vi "File Attachment Example.vi"() -> ()   [LabVIEW 2024]
uses:
  Sift API/Sift Client.lvclass
  Sift API/Types/Entity Type.ctl
  Sift Client.lvlib
panel:
  in  "Run Name":string
  out "Error":errorcluster
  in  "API Key":string
  in  "API URL":string
  # "Sift File Attachment Upload Example"
  # "Note: This example will not run as-is. \nOpen the VI to update the pathnames to valid files to run the example."
  # "Run this example to test uploading file attachments files to Sift."
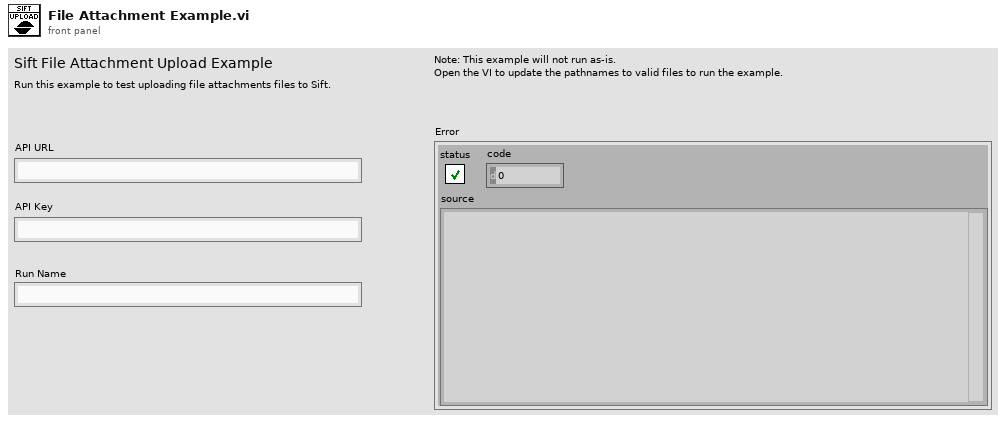
[diagram p1: front panel]
types:
  T1 = typedef "Sift Client.lvlib/Entity Type.ctl" = enum16{"runs", "annotations", "annotation_logs"}
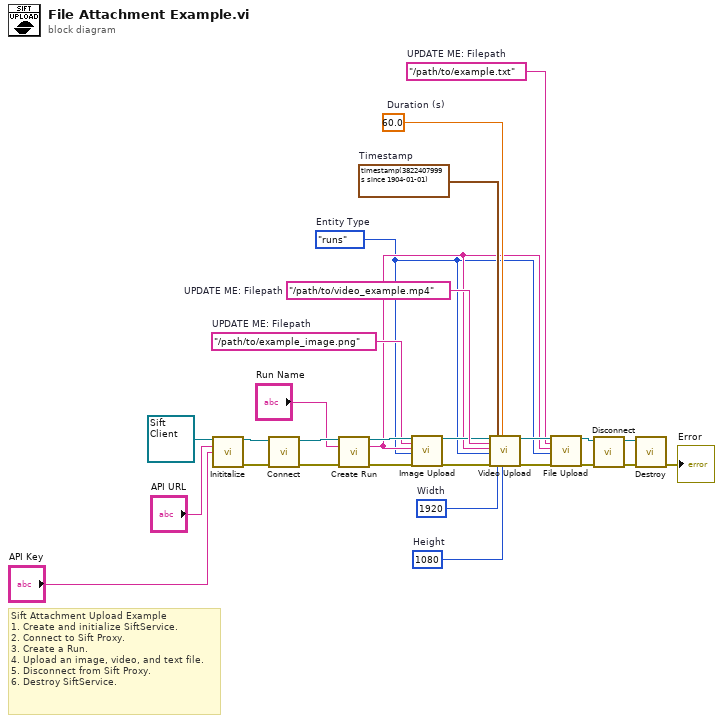
[diagram p0: block diagram]
diagram:
  w1 = "/path/to/example.txt"  # UPDATE ME: Filepath
  w8 = "/path/to/example_image.png"  # UPDATE ME: Filepath
  w13 = timestamp(3822408000.0 s since 1904-01-01)  # Timestamp
  w14 = 60.0  # Duration (s)
  w15 = 1080  # Height
  w16 = 1920  # Width
  w17 = "/path/to/video_example.mp4"  # UPDATE ME: Filepath
  w2 = Entity_Type."runs"  # Entity Type
  # "Sift Attachment Upload Example\n1. Create and initialize SiftService.\n2. Connect to Sift Proxy.\n3. Create a Run.\n4. Upload an image, video, and text file.\n5. Disconnect from Sift Proxy.\n6. Destroy SiftService."
  n1 = call-dynamic "Inititalize.vi"("Sift Client in"=refnum<class "Sift Client.lvclass"> refnum ("Sift Client.lvlib:Sift Client.lvclass"), "API URL"="API URL", "API Key"="API Key") -> ("Sift Client out"=w24:refnum<class "Sift Client.lvclass">, "error out"=w23:errorcluster)  [unwired: 11 in]
  n2 = call-dynamic "Connect.vi"("error in (no error)"=w23, "Sift Client in"=w24) -> ("error out"=w19:errorcluster, "Sift Client out"=w20:refnum<class "Sift Client.lvclass">)  [unwired: 7 in, 1 out]
  n3 = call-dynamic "Create Run.vi"("Sift Client in"=w20, "Name"="Run Name", "error in (no error)"=w19) -> ("Sift Client out"=w12:refnum<class "Sift Client.lvclass">, "Run ID"=w3:string, "error out"=w10:errorcluster)  [unwired: 9 in, 1 out]
  n4 = call-dynamic "Image Upload.vi"("Sift Client in"=w12, "Filepath"=w8, "Entity ID"=w3, "Entity Type"=w2, "error in (no error)"=w10) -> ("Sift Client out"=w11:refnum<class "Sift Client.lvclass">, "error out"=w9:errorcluster)  [unwired: 13 in]
  n5 = call-dynamic "Video Upload.vi"("Sift Client in"=w11, "Filepath"=w17, "Entity ID"=w3, "Entity Type"=w2, "error in (no error)"=w9, "Timestamp"=w13, "Width"=w16, "Duration (s)"=w14, "Height"=w15) -> ("Sift Client out"=w5:refnum<class "Sift Client.lvclass">, "error out"=w7:errorcluster)  [unwired: 9 in]
  n6 = call-dynamic "File Upload.vi"("Sift Client in"=w5, "Filepath"=w1, "Entity ID"=w3, "Entity Type"=w2, "error in (no error)"=w7) -> ("Sift Client out"=w4:refnum<class "Sift Client.lvclass">, "error out"=w6:errorcluster)  [unwired: 13 in]
  n7 = call-dynamic "Disconnect.vi"("error in (no error)"=w6, "Sift Client in"=w4) -> ("error out"=w21:errorcluster, "Sift Client out"=w22:refnum<class "Sift Client.lvclass">)  [unwired: 8 in]
  n8 = call-dynamic "Destroy.vi"("error in (no error)"=w21, "Sift Client in"=w22) -> ("error out"=→"Error":errorcluster)  [unwired: 8 in, 1 out]
